vi "Read VISA Resource.vi"(8 "error in":errorcluster, 11 "Serial Session in":refnum<class "Serial Session.lvclass">) -> (0 "error out":errorcluster, 2 "VISA Resource":refnum<visa-resource-name>, 3 "Serial Session out":refnum<class "Serial Session.lvclass">)   [LabVIEW 2016, in "Serial Session.lvclass"]
doc: "Retrieve the VISA session from the class."
uses:
  Serial Session.lvclass
  Serial Session.lvclass/Serial Session.ctl
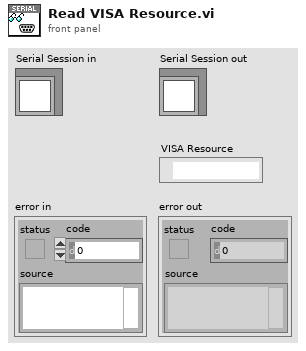
[diagram p1: front panel]
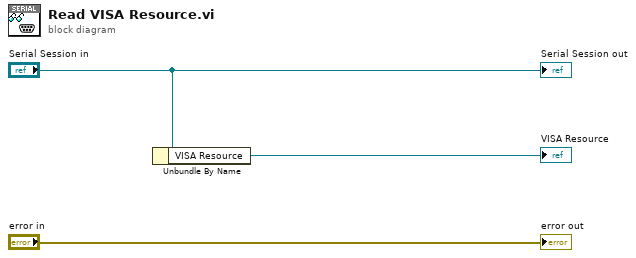
[diagram p0: block diagram]
diagram:
  n1 = Unbundle By Name("Serial Session in") -> ("VISA Resource"=→"VISA Resource":refnum<visa-resource-name>)
  "error out" <- "error in"
  "Serial Session out" <- "Serial Session in"
